vi "字符转十六进制字符串.vi"(11 "字符串输入":string) -> (3 "字符串输出":string)   [LabVIEW 2016, in "数据传输系统.lvlib"]
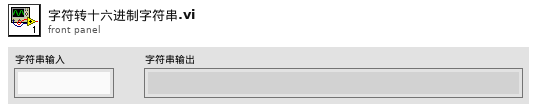
[diagram p1: front panel]
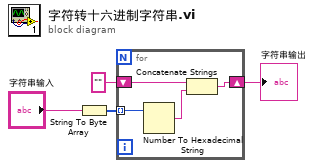
[diagram p0: block diagram]
diagram:
  n1 = String To Byte Array(string="字符串输入") -> (unsigned byte array=w2:u8[])
  n2 = for {
    tunnel: w2 -> [w8] mode=indexing
    shift-right: [w5] -> w4
    shift-left: "" -> [w6]
    n3 = Number To Hexadecimal String(2:w8) -> (0:w7:string)  [unwired: 1 in]
    n4 = Concatenate Strings(w6, w7) -> (w5:string)
  }
  "字符串输出" <- w4
